vi "Str2DBL.vi"(5 "Error Locator":string, 6 "error in (no error)":errorcluster, 8 "Current Variable settings":T1[](array[typedef]), 9 "formula":string) -> (0 "error out":errorcluster, 3 "y value":dbl)   [LabVIEW 2013]
doc: "Convert string to DBL. First try parsing with LuaVIEW \"Evaluate f(x)\", then scan for \"SI\" notation (e.g. 10u = 10e-5). Only white-space remainders allowed after the scan, otherwise an error is thrown. Output can be converted to boolean with \"!=0?\" comparison."
uses:
  TypeDefs/Active procedure variables.ctl
  <vilib>/Utility/error.llb/DialogType.ctl
panel:
  out "(Remainder String)":string
  out "(error lua)":errorcluster
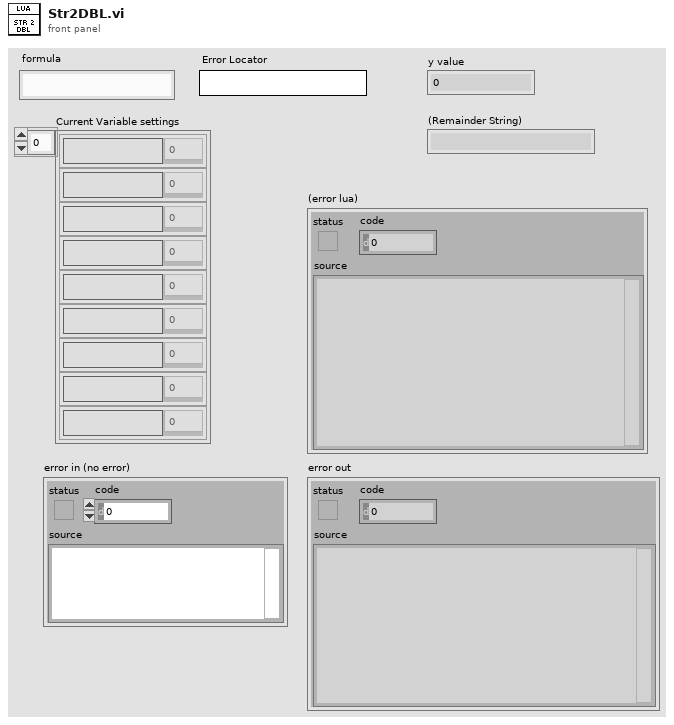
[diagram p1: front panel]
types:
  T1 = typedef "Active procedure variables.ctl" = cluster{"Procedure variable":string, "Value":dbl}
  T2 = typedef "DialogType.ctl" = u16
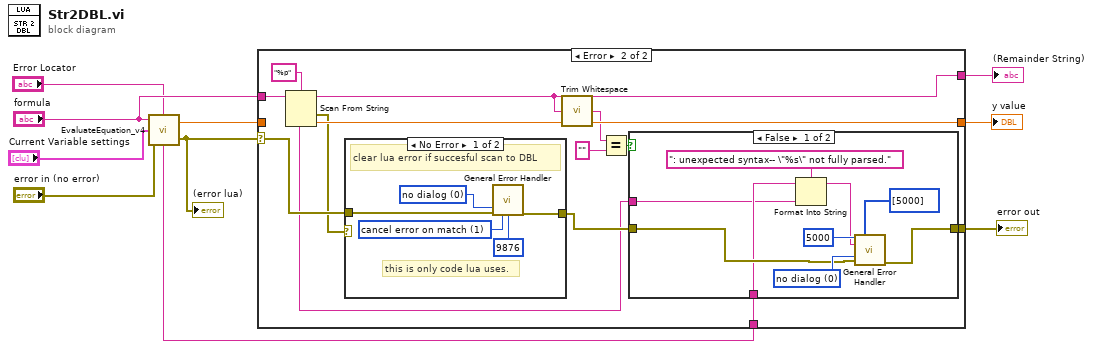
[diagram p0: block diagram]
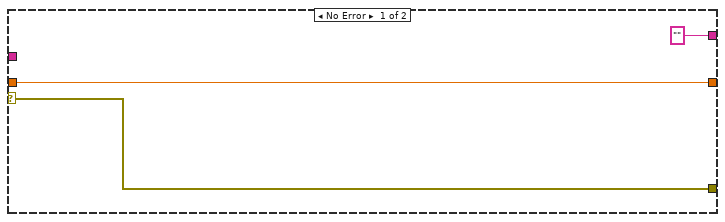
[diagram p2: hidden frame]
diagram:
  n1 = call "EvaluateEquation_v4.vi"("Error Locator"="Error Locator", "error in (no error)"="error in (no error)", "Current Variable settings"="Current Variable settings", "formula"="formula") -> ("error out"=w7:errorcluster, "y value"=w5:dbl)
  "(error lua)" <- w7
  n2 = case shown="Error" w7 {
    selector: w7 -> [w11 w22]
    tunnel: [w12 w23] -> w6
    tunnel: w5 -> [w12 _]
    tunnel: "formula" -> [_ w15]
    tunnel: [w11 w17] -> w3
    tunnel: "Error Locator" -> [_ w16]
    tunnel: ["" w13] -> w1
    frame No Error {
    }
    frame Error {
      n3 = Scan From String(format string="%p", input string=w15) -> (remaining string=w13:string, error out=w21:errorcluster, output 1=w23:dbl)  [unwired: 3 in, 1 out]
      n4 = case shown="No Error" w21 {
        tunnel: w22 -> [w39 w40]
        tunnel: [w38 w40] -> w18
        frame No Error {
          w35 = T2 0 items=["no dialog", "OK message", "continue or stop message", "OK message + warnings", "continue/stop + warnings"] ("type of dialog (OK msg:1)")
          w36 = 1 items=["no exception", "cancel error on match", "set error on match"] ("[exception action] (none:0)")
          # "this is only code lua uses."
          # "clear lua error if succesful scan to DBL"
          n5 = call <vilib>:"General Error Handler.vi"("type of dialog (OK msg:1)"=w35, "error in (no error)"=w39, "[exception action] (none:0)"=w36, "[exception code]"=9876) -> ("error out"=w38:errorcluster)  [unwired: 7 in, 4 out]
        }
        frame Error {
        }
      }
      n6 = call <vilib>:"Trim Whitespace.vi"("string"=w13) -> ("trimmed string"=w14:string)  [unwired: 1 in]
      n7 = Equal?(x=w14, y="") -> (x = y?=w19:bool)
      n8 = case shown="False" w19 {
        tunnel: w18 -> [w30 w34]
        tunnel: [w33 w34] -> w17
        tunnel: w16 -> [w28 _]
        tunnel: w15 -> [w25 _]
        frame False {
          w32 = T2 0 items=["no dialog", "OK message", "continue or stop message", "OK message + warnings", "continue/stop + warnings"] ("type of dialog (OK msg:1)")
          n9 = Format Into String(format string=": unexpected syntax-- \"%s\" not fully parsed.", initial string=w28, w25) -> (resulting string=w27:string)  [unwired: 1 in, 1 out]
          n10 = call <vilib>:"General Error Handler.vi"("[error code] (0)"=5000, "[user-defined codes]"=i32[] [5000], "[error source] (\" \")"=w27, "type of dialog (OK msg:1)"=w32, "error in (no error)"=w30) -> ("error out"=w33:errorcluster)  [unwired: 6 in, 4 out]
        }
        frame True {
        }
      }
    }
  }
  "y value" <- w6
  "error out" <- w3
  "(Remainder String)" <- w1
